vi "ForceTorqueSensor_RTL.vi"() -> ()   [LabVIEW 2019]
uses:
  <vilib>/Platform/TimedLoop/XDataNode/timing_clust.ctl
  <vilib>/Platform/TimedLoop/XDataNode/nitl_modes.ctl
  <vilib>/Platform/TimedLoop/XDataNode/wakeup.ctl
  <vilib>/Analysis/baseanly.llb/Real Dot Product.vi
  <vilib>/Utility/file.llb/Write Delimited Spreadsheet (DBL).vi
  <vilib>/platform/TimedLoop/XDataNode/XDataNode.xnode
  <vilib>/Utility/Variable/NI_VariableUtilities.lvlib
  <vilib>/Platform/TimedLoop/XDataNode/XDNodeRunTimeDep.lvlib
  <vilib>/Analysis/NI_AALBase.lvlib
panel:
  out "N":i32
  out "i":i32
  out "acquisition finished late":bool
  in  "BiasVector":path
  out "Writing Data":bool
  out "Time Stamp":timestamp
  out "Acq Polling Loop\n Finished late":bool
  out "error out 3":errorcluster
  out "loop calling state":bool
  in  "MxData":path
  out "Mx":dbl[](graph) caption="Mx ="
  out "Cdb_Mx":dbl[](array[numeric])
  out "Bias Calc Finished Late":bool
  out "N":dbl
  out "Bias Vector":dbl[](array[numeric])
  in  "Frequency (Hz)":dbl
  in  "Run Time (s)":dbl
  in  "FxData":path
  out "Cdb_Fx":dbl[](array[numeric])
  out "Fx":dbl[](graph) caption="Fx ="
  in  "Unbias":bool
  in  "Bias":bool
  out "Voltages":dbl[][](array[numeric])
  in  "Guage Data":path
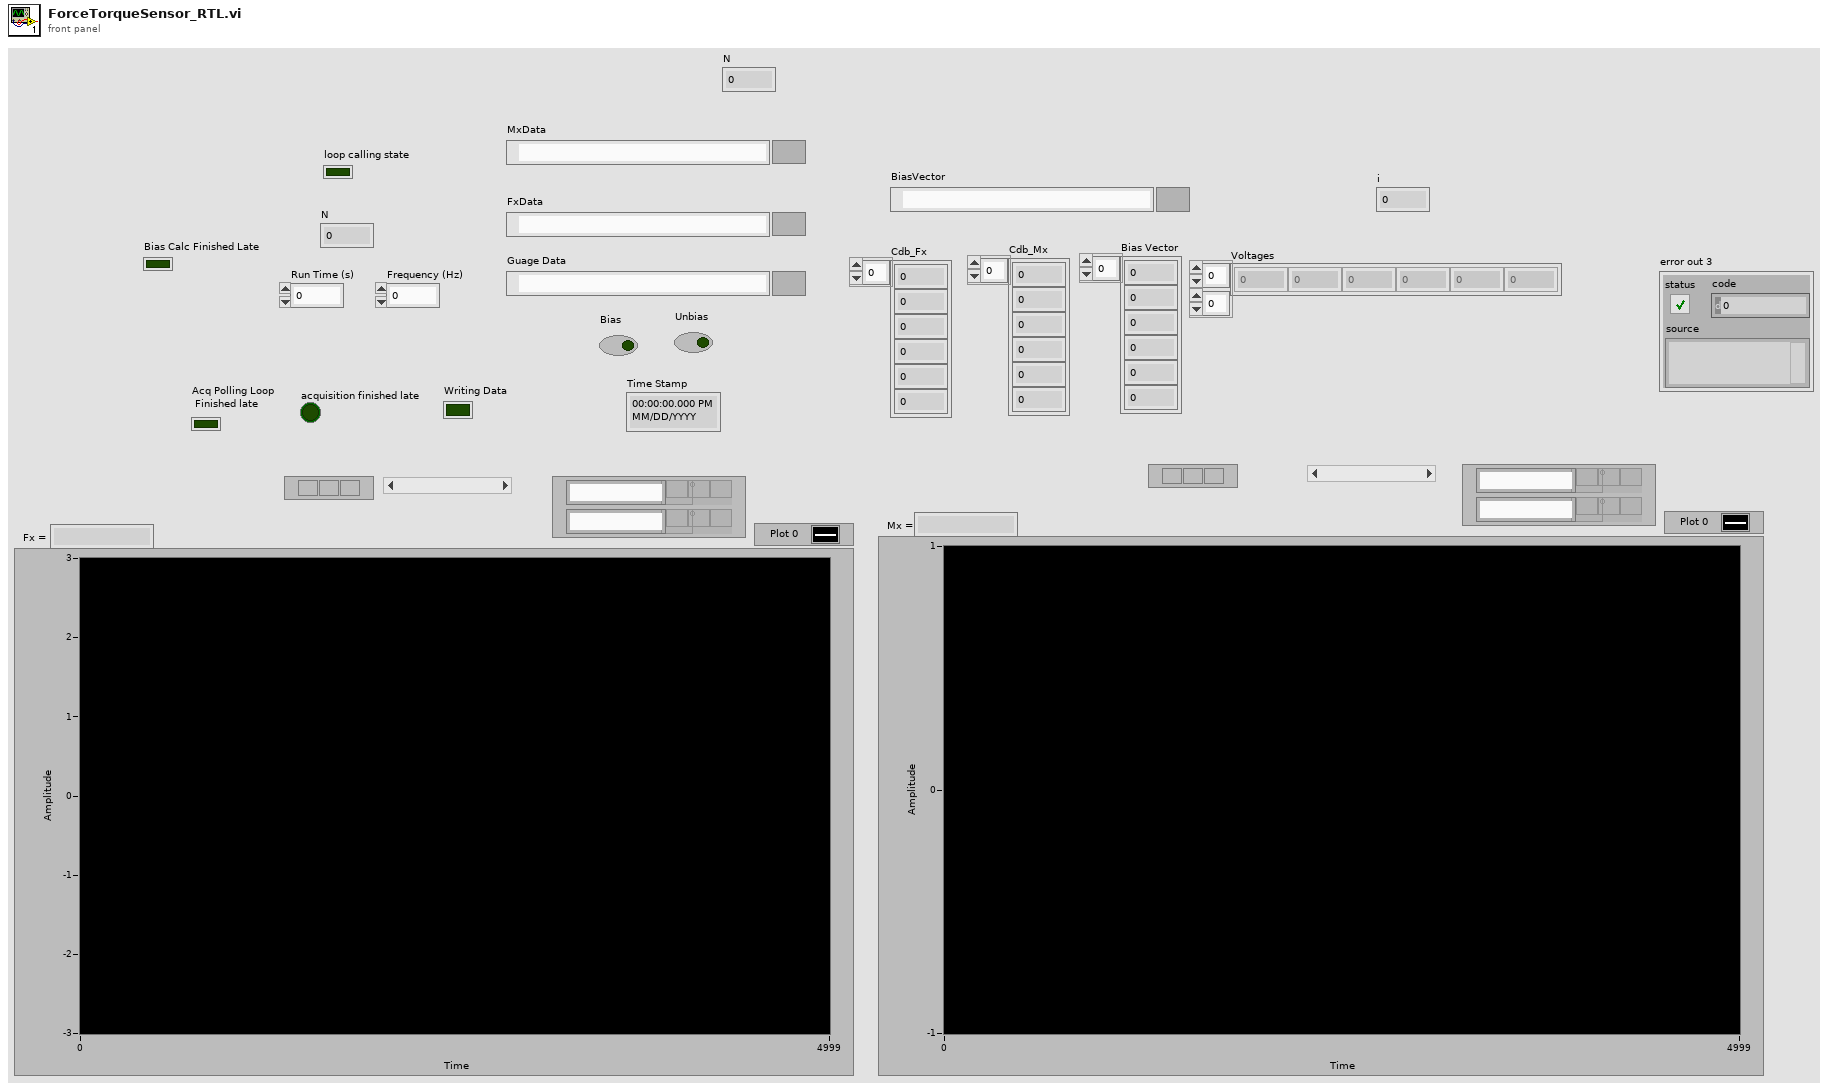
[diagram p1: front panel]
types:
  T1 = typedef "XDNodeRunTimeDep.lvlib/timing_clust.ctl" = cluster{"Expected End [f-1]":u64, "Actual End [f-1]":u64, "Finished Late? [f-1]":bool, "Expected End [i-1]":u64, "Actual End [i-1]":u64, "Finished Late? [i-1]":bool, "Expected Start [i]":u64, "Actual Start [i]":u64, "Expected Start [f]":u64, "Actual Start [f]":u64, "Source Name":string, "Structure Name":string, "Period":i64, "Deadline":i64, "Offset":i64, "Start":i64, "Priority":i32, "Timeout":i32, "Mode":T2, "Wakeup Reason":T3, "Error":errorcluster, "Source Type":string, "Secondary Source Type":string, "Global End Time":u64, "Global Start Time":u64, "Frame Duration":u64, "Iteration Duration":u64, "Assigned CPU":i32, "I/O Scan Engine Mode":u32}
  T2 = typedef "XDNodeRunTimeDep.lvlib/nitl_modes.ctl" = enum32{"No Change", "Process missed periods, maintain original phase", "Discard missed periods, maintain original phase", "Process missed periods, ignore original phase", "Discard missed periods, ignore original phase"}
  T3 = typedef "XDNodeRunTimeDep.lvlib/wakeup.ctl" = enum32{"Normal", "Aborted", "Asynchronous wakeup", "Timing source error", "Timed loop error", "Timeout"}
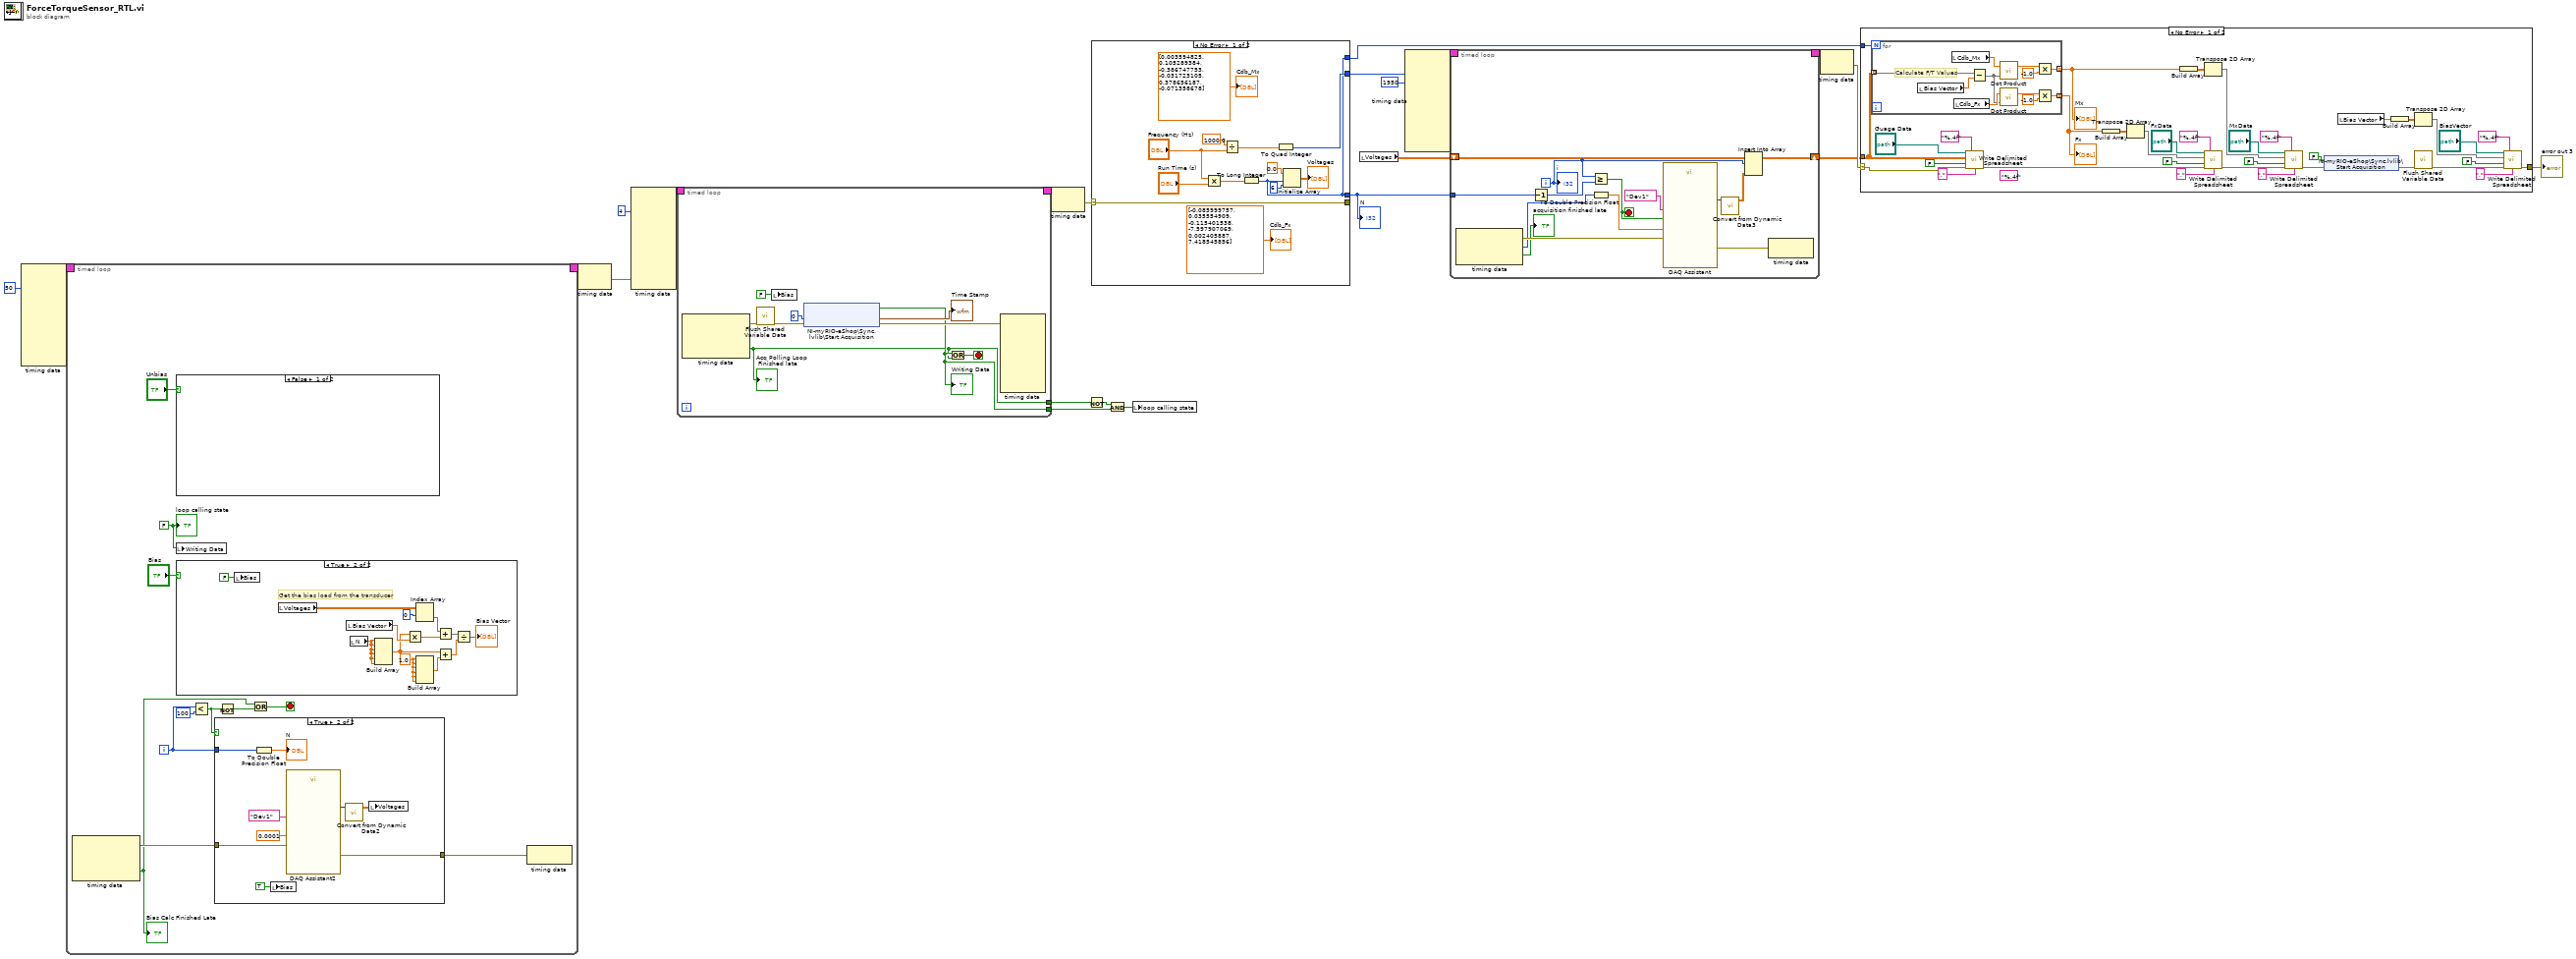
[diagram p0: block diagram]
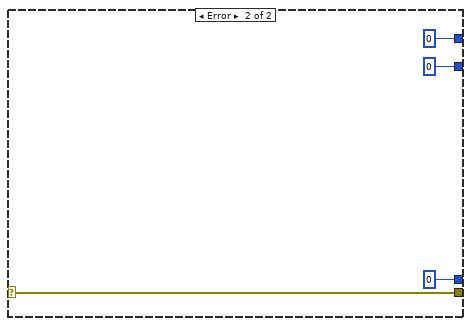
[diagram p2: hidden frame]
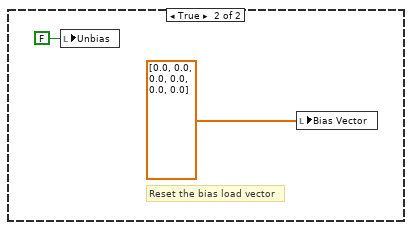
[diagram p5: hidden frame]
diagram:
  n1 = node-c288(i64 50 ("Period")) -> (w22:T1)  [unwired: 9 in]
  n2 = timed-loop {
    timing: w22 -> [_]
    timing-out: [_] -> w21
    i -> [w30]
    stop <- w27 stop-if-true
    w23 = FALSE ("loop calling state")
    n3 = node-c288() -> (w26:errorcluster, w24:bool)  [unwired: 1 in, 2 out]
    "Bias Calc Finished Late" <- w24
    n4 = case shown="False" "Unbias" {
      frame False {
      }
      frame True {
        # "Reset the bias load vector"
        n5 = local write "Unbias"(FALSE) -> ()
        n6 = local write "Bias Vector"(dbl[] [0.0, 0.0, 0.0, 0.0, 0.0, 0.0]) -> ()
      }
    }
    n7 = local write "Writing Data"(w23) -> ()
    n8 = case shown="True" "Bias" {
      frame False {
      }
      frame True {
        w51 = 1.0 ("element")
        # "Get the bias load from the transducer"
        n9 = local write "Bias"(FALSE) -> ()
        n10 = local read "Voltages"() -> (w58:dbl[][])
        n11 = local read "Bias Vector"() -> (w54:dbl[])
        n12 = local read "N"() -> (w55:dbl)
        n13 = Build Array(w55, w55, w55, w55, w55, w55) -> (w49:dbl[])
        n14 = Multiply(x=w49, y=w54) -> (x*y=w52:dbl[])
        n15 = Index Array(array=w58, index (row)=0) -> (element=w53:dbl[])  [unwired: 1 in]
        n16 = Build Array(w51, w51, w51, w51, w51, w51) -> (w50:dbl[])
        n17 = Add(x=w53, y=w52) -> (x+y=w46:dbl[])
        n18 = Add(x=w49, y=w50) -> (x+y=w47:dbl[])
        n19 = Divide(x=w46, y=w47) -> (x/y=→"Bias Vector":dbl[])
      }
    }
    n20 = Less?(x=w30, y=100) -> (x < y?=w29:bool)
    n21 = case shown="True" w29 {
      tunnel: w30 -> [_ w38]
      tunnel: w26 -> [w34 w36]
      tunnel: [w34 w35] -> w25
      frame False {
      }
      frame True {
        n22 = To Double Precision Float(number=w38) -> (double precision float=→"N":dbl)
        n23 = local write "Bias"(TRUE) -> ()
        n24 = call "DAQ Assistant2"("timeout (s)"=0.0001, "error in"=w36, "device name"=tag "Dev1") -> ("data"=w40:dynamicdata, "error out"=w35:errorcluster)  [unwired: 14 in, 1 out]
        n25 = call "Convert from Dynamic Data2"("Dynamic Data Type"=w40) -> ("Array"=w39:dbl[][])  [unwired: 3 in]
        n26 = local write "Voltages"(w39) -> ()
      }
    }
    n27 = Not(x=w29) -> (.not. x?=w28:bool)
    n28 = Or(x=w24, y=w28) -> (x .or. y?=w27:bool)
    n29 = node-c288(w25) -> ()  [unwired: 1 out]
    "loop calling state" <- w23
  }
  n30 = node-c288(w21) -> (w6:errorcluster)
  n31 = node-c288(i64 4 ("Period"), w6) -> (w12:T1)  [unwired: 8 in]
  n32 = timed-loop {
    timing: w12 -> [_]
    timing-out: [_] -> w11
    tunnel: [w67] -> w9
    tunnel: [w66] -> w7
    stop <- w68 stop-if-true
    n33 = node-c288() -> (w71:errorcluster, w66:bool)  [unwired: 1 in, 2 out]
    "Acq Polling Loop\n Finished late" <- w66
    n34 = call <vilib>:"Flush Shared Variable Data.vi"("error in (no error)"=w71) -> ("error out"=w70:errorcluster)  [unwired: 10 in]
    n35 = local write "Bias"(FALSE) -> ()
    n36 = shared-variable "NI-myRIO-eShop\\Sync.lvlib\\Start Acquisition"(error in=w70, 0 ("ms timeout (0)")) -> (w67:bool, error out=w69:errorcluster, →"Time Stamp":timestamp)  [unwired: 1 out]
    "Writing Data" <- w67
    n37 = Or(x=w67, y=w66) -> (x .or. y?=w68:bool)
    n38 = node-c288(w69) -> ()  [unwired: 7 in, 1 out]
  }
  n39 = node-c288(w11) -> (w4:errorcluster)
  n40 = Not(x=w7) -> (.not. x?=w8:bool)
  n41 = case shown="No Error" w4 {
    selector: w4 -> [w83 w96]
    tunnel: [w82 0] -> w16
    tunnel: [w84 i64 0] -> w15
    tunnel: [w83 w96] -> _
    tunnel: [w82 0] -> w14
    frame No Error {
      n42 = Multiply(x="Frequency (Hz)", y="Run Time (s)") -> (x*y=w89:dbl)
      n43 = Divide(x=1000.0, y="Frequency (Hz)") -> (x/y=w85:dbl)
      n44 = To Long Integer(number=w89) -> (32bit integer=w82:i32)
      n45 = To Quad Integer(1:w85) -> (0:w84:i64)
      n46 = Initialize Array(0.0 ("element"), w82, 6 ("dimension size")) -> (→"Voltages":dbl[][])
      "Cdb_Fx" <- dbl[] [-0.085999757, 0.035554909, -0.115401538, -7.597907069, 0.002405887, 7.418545856]
      "Cdb_Mx" <- dbl[] [0.003594825, 0.105289384, -0.386747753, -0.031723105, 0.378656187, -0.071358678] ("Cdb 2")
    }
    frame Error {
    }
  }
  "N" <- w14
  n47 = And(x=w8, y=w9) -> (x .and. y?=w5:bool)
  n48 = local write "loop calling state"(w5) -> ()
  n49 = local read "Voltages"() -> (w3:dbl[][])
  n50 = node-c288(w15, 1950 ("Priority")) -> (w18:T1)  [unwired: 8 in]
  n51 = timed-loop {
    timing: w18 -> [_]
    timing-out: [_] -> w17
    tunnel: w14 -> [w103]
    shift-right: [w100] -> w2
    shift-left: w3 -> [w101]
    i -> [w99]
    stop <- w102 stop-if-true
    n52 = node-c288() -> (w107:errorcluster, w104:i64, →"acquisition finished late":bool)  [unwired: 1 in]
    n53 = Decrement(x=w103) -> (x-1=w97:i32)
    n54 = Greater Or Equal?(x=w99, y=w97) -> (x >= y?=w102:bool)
    n55 = To Double Precision Float(number=w104) -> (double precision float=w105:dbl)
    n56 = call "DAQ Assistant"("timeout (s)"=w105, "error in"=w107, "stop (T)"=w102, "device name"=tag "Dev1") -> ("data"=w109:dynamicdata, "error out"=w106:errorcluster)  [unwired: 13 in, 1 out]
    n57 = call "Convert from Dynamic Data3"("Dynamic Data Type"=w109) -> ("Array"=w108:dbl[][])  [unwired: 3 in]
    n58 = Insert Into Array(array=w101, index (row)=w99, new element=w108) -> (w100:dbl[][])  [unwired: 1 in]
    n59 = node-c288(w106) -> ()  [unwired: 1 out]
    "i" <- w99
  }
  n60 = node-c288(w17) -> (w13:errorcluster)
  n61 = case shown="No Error" w13 {
    selector: w13 -> [w130 w164]
    tunnel: [w119 w164] -> w19
    tunnel: w16 -> [w132 _]
    tunnel: w2 -> [w131 _]
    frame No Error {
      (unwired) "%.4f" ("format (%.3f)")
      n62 = for {
        N: w132 -> [_]
        tunnel: w131 -> [w163] mode=indexing
        tunnel: [w160] -> w146 mode=indexing
        tunnel: [w153] -> w135 mode=indexing
        # "Calculate F/T Values"
        n63 = local read "Bias Vector"() -> (w162:dbl[])
        n64 = local read "Cdb_Mx"() -> (w155:dbl[])
        n65 = local read "Cdb_Fx"() -> (w161:dbl[])
        n66 = Subtract(x=w163, y=w162) -> (x-y=w154:dbl[])
        n67 = call-poly <vilib>:"Dot Product.vi"("Y Vector"=w154, "X Vector"=w155) -> ("X * Y"=w157:dbl)  [unwired: 1 out]
        n68 = call-poly <vilib>:"Dot Product.vi"("Y Vector"=w154, "X Vector"=w161) -> ("X * Y"=w159:dbl)  [unwired: 1 out]
        n69 = Multiply(x=w157, y=-1.0) -> (x*y=w153:dbl)
        n70 = Multiply(x=w159, y=-1.0) -> (x*y=w160:dbl)
      }
      "Fx" <- w146
      "Mx" <- w135
      n71 = call-poly <vilib>:"Write Delimited Spreadsheet.vi"("file path (dialog if empty)"="Guage Data", "format (%.3f)"="%.4f", "2D data"=w131, "append to file? (new file:F)"=FALSE, "error in (no error)"=w130, "delimiter (\\t)"="," ("delimiter (\\t)")) -> ("error out"=w134:errorcluster)  [unwired: 8 in, 1 out]
      n72 = Build Array(w146) -> (w145:dbl[][])
      n73 = Transpose 2D Array(2D array=w145) -> (transposed array=w144:dbl[][])
      n74 = Build Array(w135) -> (w138:dbl[][])
      n75 = Transpose 2D Array(2D array=w138) -> (transposed array=w137:dbl[][])
      n76 = call-poly <vilib>:"Write Delimited Spreadsheet.vi"("file path (dialog if empty)"="FxData", "format (%.3f)"="%.4f", "2D data"=w144, "append to file? (new file:F)"=FALSE, "error in (no error)"=w134, "delimiter (\\t)"="," ("delimiter (\\t)")) -> ("error out"=w136:errorcluster)  [unwired: 8 in, 1 out]
      n77 = call-poly <vilib>:"Write Delimited Spreadsheet.vi"("file path (dialog if empty)"="MxData", "format (%.3f)"="%.4f", "2D data"=w137, "append to file? (new file:F)"=FALSE, "error in (no error)"=w136, "delimiter (\\t)"="," ("delimiter (\\t)")) -> ("error out"=w133:errorcluster)  [unwired: 8 in, 1 out]
      n78 = shared-variable "NI-myRIO-eShop\\Sync.lvlib\\Start Acquisition"(FALSE ("Start Acquisition"), error in=w133) -> (error out=w142:errorcluster)
      n79 = local read "Bias Vector"() -> (w121:dbl[])
      n80 = Build Array(w121) -> (w124:dbl[][])
      n81 = Transpose 2D Array(2D array=w124) -> (transposed array=w123:dbl[][])
      n82 = call <vilib>:"Flush Shared Variable Data.vi"("error in (no error)"=w142) -> ("error out"=w120:errorcluster)  [unwired: 10 in]
      n83 = call-poly <vilib>:"Write Delimited Spreadsheet.vi"("file path (dialog if empty)"="BiasVector", "format (%.3f)"="%.4f", "2D data"=w123, "append to file? (new file:F)"=FALSE, "error in (no error)"=w120, "delimiter (\\t)"="," ("delimiter (\\t)")) -> ("error out"=w119:errorcluster)  [unwired: 8 in, 1 out]
    }
    frame Error {
    }
  }
  "error out 3" <- w19
